vi "VL Type.vi"(8 "error in (no error)":errorcluster, 11 "Node in":refnum<class "Node.lvclass">) -> (0 "error out":errorcluster, 2 "VL Type":T1, 3 "Node out":refnum<class "Node.lvclass">)   [LabVIEW 2020, in "VolatusConfig.lvlib" / "Node.lvclass"]
uses:
  Node.lvclass
  Meta Type.ctl
  Node.lvclass/Node.ctl
  VolatusConfig.lvlib
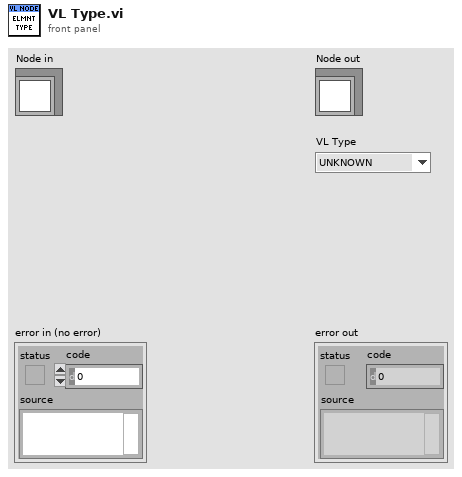
[diagram p1: front panel]
types:
  T1 = typedef "VolatusConfig.lvlib/Meta Type.ctl" = enum16{"UNKNOWN", "VL_System", "VL_Cluster", "VL_Node", "VL_Task", "VL_Group", "VL_Channel", "VL_Task_List", "VL_Scaling"}
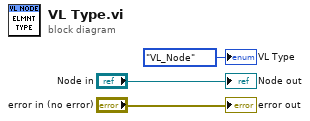
[diagram p0: block diagram]
diagram:
  "error out" <- "error in (no error)"
  "Node out" <- "Node in"
  "VL Type" <- Meta_Type."VL_Node" ("VL Type")
